vi "sequenced_structure.vi"() -> ()   [LabVIEW 2012]
panel:
  out "string_indicator":string
  in  "string_control":string
  in  "stop 2":bool
  in  "stop":bool
  out "frame 1":string
  out "frame 2":string
  out "numeric_ indicator":dbl
  in  "numeric_control":dbl
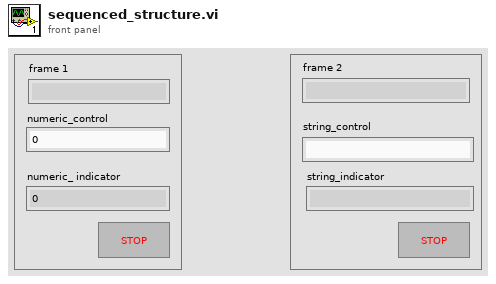
[diagram p1: front panel]
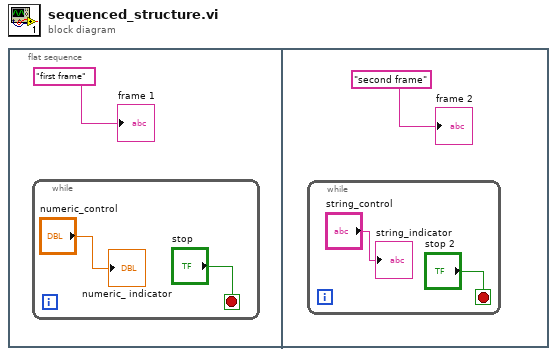
[diagram p0: block diagram]
diagram:
  n1 = flat-sequence {
    frame #0 {
      n2 = while {
        stop <- "stop" stop-if-true
        "numeric_ indicator" <- "numeric_control"
      }
      "frame 1" <- "first frame"
    }
    frame #1 {
      n3 = while {
        stop <- "stop 2" stop-if-true
        "string_indicator" <- "string_control"
      }
      "frame 2" <- "second frame"
    }
  }
